vi "Write Wash Display Console.vi"(8 "error in (no error)":errorcluster, 10 "Architecture.lvlib:Queue.lvclass":refnum<class "Queue.lvclass">, 11 "Car Wash Controller in":refnum<class "Car Wash Controller.lvclass">) -> (0 "error out":errorcluster, 3 "Car Wash Controller out":refnum<class "Car Wash Controller.lvclass">)   [LabVIEW 2012, in "Car Wash Controller.lvlib" / "Car Wash Controller.lvclass"]
uses:
  Car Wash Controller.lvclass
  Queue/Queue.lvclass
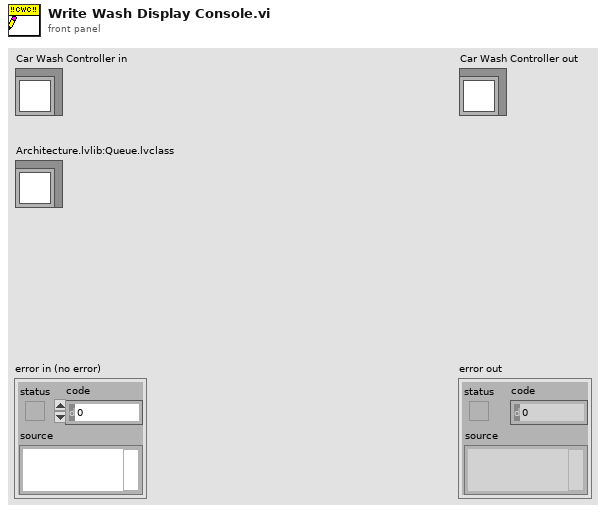
[diagram p1: front panel]
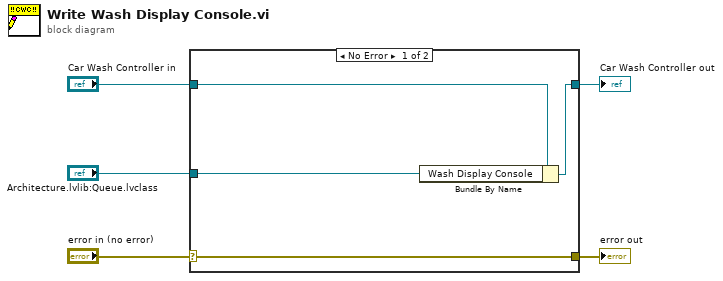
[diagram p0: block diagram]
diagram:
  n1 = case shown="No Error" "error in (no error)" {
    selector: "error in (no error)" -> [w9 w10]
    tunnel: [w9 w10] -> w4
    tunnel: [w7 w11] -> w2
    tunnel: "Car Wash Controller in" -> [w8 w11]
    tunnel: "Architecture.lvlib:Queue.lvclass" -> [w6 _]
    frame No Error {
      n2 = Bundle By Name(cluster=w8, "Wash Display Console"=w6) -> (w7:refnum<class "Car Wash Controller.lvclass">)
    }
    frame Error {
    }
  }
  "error out" <- w4
  "Car Wash Controller out" <- w2
